vi "TestStand, Set Step Name.vi"(8 "error in":errorcluster, 10 "Step Name":string="Sequence Step General: Name", 11 "Sequence Context":refnum<k7>) -> (0 "error out":errorcluster, 3 "Sequence Context Out":refnum<k7>)   [LabVIEW 2010]
doc: "This function sets the TestStand Sequence step name. The step name will appear on the test report instead of the TestStand Sequence Step General Tab name field."
uses:
  <vilib>/addons/TestStand/_TSUtility.llb/TestStand - Get Property Value (Object).vi
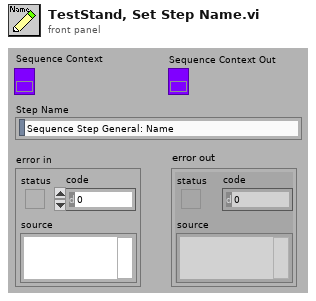
[diagram p1: front panel]
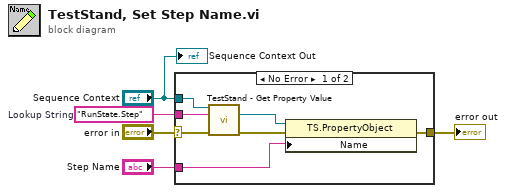
[diagram p0: block diagram]
diagram:
  w1 = "RunState.Step"  # Lookup String
  n1 = case shown="No Error" "error in" {
    selector: "error in" -> [w8 w13]
    tunnel: [w9 w13] -> w5
    tunnel: "Sequence Context" -> [w10 _]
    tunnel: "Step Name" -> [w7 _]
    tunnel: w1 -> [w6 _]
    frame No Error {
      n2 = call-poly <vilib>:"TestStand - Get Property Value.vi"("Sequence Context In"=w10, "Lookup String"=w6, "error in (no error)"=w8) -> ("Value"=w12:refnum<k7>, "error out"=w11:errorcluster)  [unwired: 10 in, 1 out]
      n3 = property class="TS.PropertyObject"(reference=w12, error in=w11, "Name"=w7) -> (error out=w9:errorcluster)  [unwired: 1 out]
    }
    frame Error {
    }
  }
  "error out" <- w5
  "Sequence Context Out" <- "Sequence Context"
